vi "Find ROI Max Location v2.vi"(8 "error in (no error)":errorcluster, 9 "Source Image ROI Mask":T1, 10 "Source Image":T1, 11 "ROI Descriptor in":T2 {"Contours"."Type" items=["No Selection", "Point", "Line", "Rectangle", "Oval", "Polygon", "Freehand Region", "Annulus", "Unused2", "Unused3", "Broken Line", "Freehand Line", "Rotated Rectangle"]}) -> (0 "error out":errorcluster, 1 "Height":i32, 2 "Width":i32, 3 "ROI Mean Max Location":cluster{"X":i32, "Y":i32})   [LabVIEW 2021, in "Image.lvlib"]
uses:
  Image.lvlib
  <vilib>/vision/Image Controls.llb/IMAQ Image.ctl
  <vilib>/vision/EDVR.llb/IMAQ ImageToEDVR 2D U8.vi
  <vilib>/vision/EDVR.llb/IMAQ ImageToEDVR 2D I16.vi
  <vilib>/vision/EDVR.llb/IMAQ ImageToEDVR 2D SGL.vi
  <vilib>/vision/EDVR.llb/IMAQ ImageToEDVR 2D U16.vi
  <vilib>/vision/NI_Vision_Development_Module.lvlib
  Error/Error.lvlib
  Arrays/Arrays.lvlib
  Time/Time.lvlib
panel:
  out "elapsed (relative) seconds":dbl
  out "Waveform Chart":dbl[][](graph)
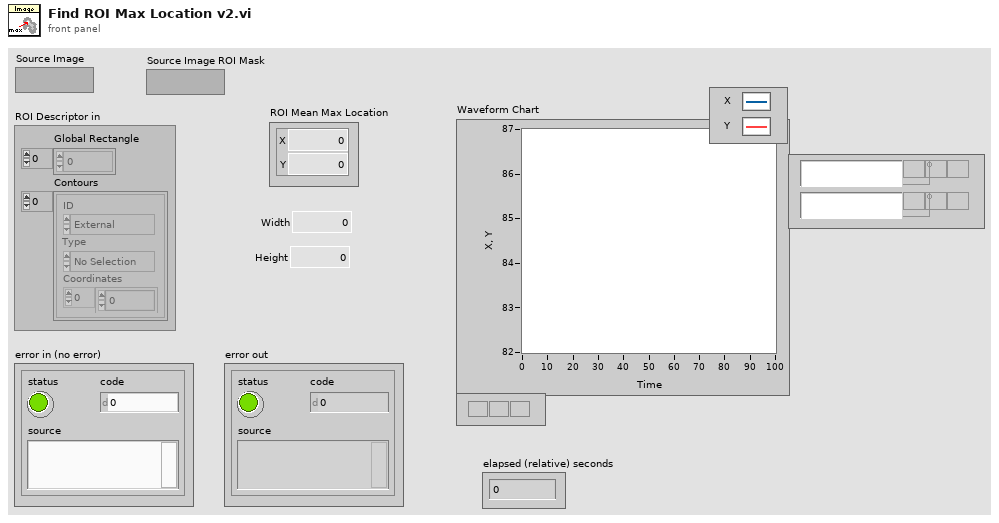
[diagram p1: front panel]
types:
  T1 = typedef "IMAQ Image.ctl" = refnum<image>
  T2 = typedef "ROI Descriptor" = cluster{"Global Rectangle":i32[], "Contours":cluster{"ID":enum32{"External", "Internal"}, "Type":u32, "Coordinates":i32[]}[]}
  T3 = typedef "Image Type" = u32
  T4 = cluster{"Numeric Control":i32, "Numeric Control":i32}[]
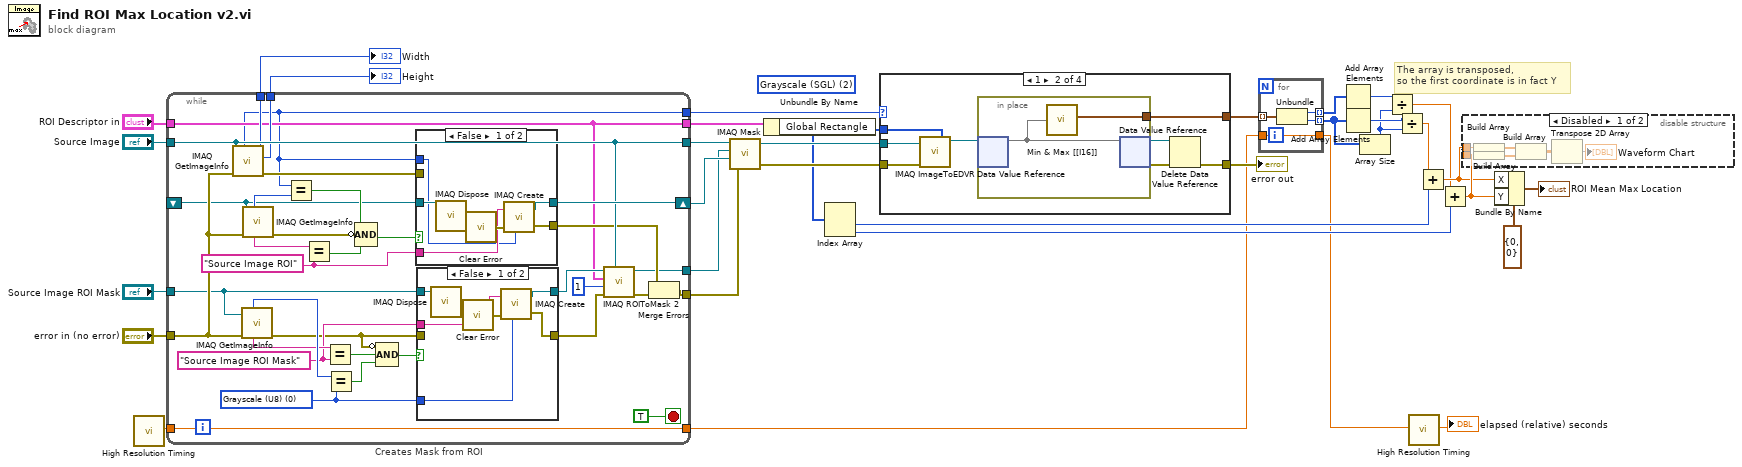
[diagram p0: block diagram]
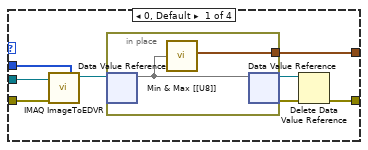
[diagram p3: hidden frame]
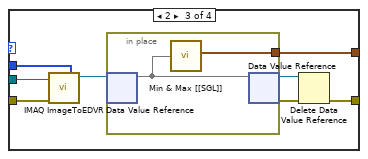
[diagram p4: hidden frame]
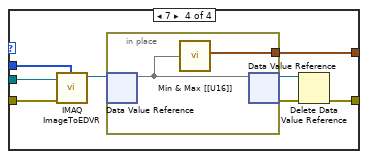
[diagram p5: hidden frame]
diagram:
  (unwired) T3 2 items=["Grayscale (U8)", "Grayscale (I16)", "Grayscale (SGL)", "Complex (CSG)", "RGB (U32)", "HSL (U32)", "RGB (U64)", "Grayscale (U16)"] ("Image Type")
  # "The array is transposed,\nso the first coordinate is in fact Y"
  n1 = call "High Resolution Timing.vi"() -> ("elapsed (relative) seconds"=w6:dbl)  [unwired: 17 in, 2 out]
  n2 = while "Creates Mask from ROI" {
    tunnel: "ROI Descriptor in" -> [w40]
    tunnel: "Source Image" -> [w47]
    tunnel: "error in (no error)" -> [w55]
    shift-right: [w49] -> w30
    shift-left: _ -> [w48]
    tunnel: [w47] -> w31
    tunnel: [w45] -> w29
    tunnel: [w42] -> w28
    tunnel: [w41] -> w27
    tunnel: [w40] -> w24
    tunnel: [w39] -> w23
    tunnel: w6 -> [w38]
    tunnel: [w38] -> w5
    tunnel: "Source Image ROI Mask" -> [w36]
    tunnel: [w35] -> w1
    stop <- TRUE stop-if-true
    w37 = "Source Image ROI" ("Image Name")
    w61 = "Source Image ROI Mask" ("Image Name")
    w60 = T3 0 items=["Grayscale (U8)", "Grayscale (I16)", "Grayscale (SGL)", "Complex (CSG)", "RGB (U32)", "HSL (U32)", "RGB (U64)", "Grayscale (U16)"] ("Image Type")
    n3 = call "IMAQ GetImageInfo"("error in (no error)"=w55, "Image"=w47) -> ("error out"=w43:errorcluster, "Y Resolution"=w41:i32, "X Resolution"=w42:i32, "Image Type"=w39:T3)  [unwired: 2 in, 4 out]
    n4 = call "IMAQ GetImageInfo"("error in (no error)"=w55, "Image"=w36) -> ("error out"=w58:errorcluster, "Image Name"=w66:string, "Image Type"=w67:T3)  [unwired: 2 in, 5 out]
    n5 = call "IMAQ GetImageInfo"("error in (no error)"=w55, "Image"=w48) -> ("error out"=w52:errorcluster, "Image Name"=w56:string, "Image Type"=w54:T3)  [unwired: 2 in, 5 out]
    n6 = Equal?(x=w39, y=w54) -> (x = y?=w51:bool)
    n7 = Equal?(x=w56, y=w37) -> (x = y?=w53:bool)
    n8 = Equal?(x=w66, y=w61) -> (x = y?=w64:bool)
    n9 = Equal?(x=w67, y=w60) -> (x = y?=w65:bool)
    n10 = Compound Arithmetic op=AND(w51, invert w52, w53) -> (w50:bool)
    n11 = Compound Arithmetic op=AND(invert w58, w64, w65) -> (w63:bool)
    n12 = case shown="False" w50 {
      tunnel: w48 -> [w75 w77]
      tunnel: w37 -> [w72 _]
      tunnel: w39 -> [w71 _]
      tunnel: [w70 w77] -> w49
      tunnel: [w69 w76] -> w44
      tunnel: w43 -> [_ w76]
      frame False {
        n13 = call "IMAQ Dispose"("Image"=w75) -> ("error out"=w74:errorcluster)  [unwired: 5 in]
        n14 = call "Clear Error.vi"("Error In"=w74) -> ("no Error Out"=w73:errorcluster)  [unwired: 8 in]
        n15 = call "IMAQ Create"("Image Name"=w72, "Image Type"=w71, "error in (no error)"=w73) -> ("New Image"=w70:T1, "error out"=w69:errorcluster)  [unwired: 2 in]
      }
      frame True {
      }
    }
    n16 = case shown="False" w63 {
      tunnel: w36 -> [w84 w86]
      tunnel: [w79 w86] -> w62
      tunnel: w61 -> [w81 _]
      tunnel: w60 -> [w80 _]
      tunnel: [w78 w85] -> w59
      tunnel: w58 -> [_ w85]
      frame False {
        n17 = call "IMAQ Dispose"("Image"=w84) -> ("error out"=w83:errorcluster)  [unwired: 5 in]
        n18 = call "Clear Error.vi"("Error In"=w83) -> ("no Error Out"=w82:errorcluster)  [unwired: 8 in]
        n19 = call "IMAQ Create"("Image Name"=w81, "Image Type"=w80, "error in (no error)"=w82) -> ("New Image"=w79:T1, "error out"=w78:errorcluster)  [unwired: 2 in]
      }
      frame True {
      }
    }
    n20 = call "IMAQ ROIToMask 2"("Image Model"=w47, "error in (no error)"=w59, "Filling Value (255)"=1, "ROI Descriptor"=w40, "Image"=w62) -> ("error out"=w46:errorcluster, "Image Out"=w35:T1)  [unwired: 4 in, 1 out]
    n21 = Merge Errors(w44, w46) -> (w45:errorcluster)
  }
  "Width" <- w28
  "Height" <- w27
  n22 = call "IMAQ Mask"("error in (no error)"=w29, "Image Dst"=w30, "Image Mask"=w1, "Image Src"=w31) -> ("error out"=w25:errorcluster, "Image Dst Out"=w26:T1)  [unwired: 1 in]
  n23 = Unbundle By Name(w24) -> ("Global Rectangle"=w22:i32[])
  n24 = Index Array(array=w22) -> (element #1=w21:i32, element #2=w20:i32)  [unwired: 2 in]
  n25 = case shown="1" w23 {
    tunnel: w26 -> [w94 w104 w114 w124]
    tunnel: w25 -> [w93 w103 w113 w123]
    tunnel: w22 -> [w92 w102 w112 w122]
    tunnel: [w90 w100 w110 w120] -> w15
    tunnel: [w87 w97 w107 w117] -> w7
    frame 0, Default {
      n26 = call-poly <vilib>:"IMAQ ImageToEDVR.vi"("Optional Rectangle"=w92, "error in (no error)"=w93, "Image"=w94) -> ("EDVR 2D U8"=w91:refnum<data-value>)  [unwired: 6 in, 2 out]
      n27 = in-place {
        in-place-border: [w96] -> w90
        n28 = in-place-dvr #1(w91) -> (w95:u8[][])  [unwired: 1 out]
        n29 = call "Min & Max [[U8]].vi"("Array"=w95) -> ("Array of Max Indices"=w96:T4)  [unwired: 4 in, 5 out]
        n30 = in-place-dvr #1(w95) -> (w89:refnum<data-value>, w88:errorcluster)
      }
      n31 = Delete Data Value Reference(data value reference=w89, error in=w88) -> (error out=w87:errorcluster)  [unwired: 1 out]
    }
    frame 1 {
      n32 = call-poly <vilib>:"IMAQ ImageToEDVR.vi"("Optional Rectangle"=w102, "error in (no error)"=w103, "Image"=w104) -> ("EDVR 2D I16"=w101:refnum<data-value>)  [unwired: 6 in, 2 out]
      n33 = in-place {
        in-place-border: [w106] -> w100
        n34 = in-place-dvr #2(w101) -> (w105:i16[][])  [unwired: 1 out]
        n35 = call "Min & Max [[I16]].vi"("Array"=w105) -> ("Array of Max Indices"=w106:T4)  [unwired: 4 in, 5 out]
        n36 = in-place-dvr #2(w105) -> (w99:refnum<data-value>, w98:errorcluster)
      }
      n37 = Delete Data Value Reference(data value reference=w99, error in=w98) -> (error out=w97:errorcluster)  [unwired: 1 out]
    }
    frame 2 {
      n38 = call-poly <vilib>:"IMAQ ImageToEDVR.vi"("Optional Rectangle"=w112, "error in (no error)"=w113, "Image"=w114) -> ("EDVR 2D SGL"=w111:refnum<data-value>)  [unwired: 6 in, 2 out]
      n39 = in-place {
        in-place-border: [w116] -> w110
        n40 = in-place-dvr #3(w111) -> (w115:sgl[][])  [unwired: 1 out]
        n41 = call "Min & Max [[SGL]].vi"("Array"=w115) -> ("Array of Max Indices"=w116:T4)  [unwired: 4 in, 5 out]
        n42 = in-place-dvr #3(w115) -> (w109:refnum<data-value>, w108:errorcluster)
      }
      n43 = Delete Data Value Reference(data value reference=w109, error in=w108) -> (error out=w107:errorcluster)  [unwired: 1 out]
    }
    frame 7 {
      n44 = call-poly <vilib>:"IMAQ ImageToEDVR.vi"("Optional Rectangle"=w122, "error out"=w123, "Image"=w124) -> ("EDVR 2D U16"=w121:refnum<data-value>)  [unwired: 6 in, 2 out]
      n45 = in-place {
        in-place-border: [w126] -> w120
        n46 = in-place-dvr #4(w121) -> (w125:u16[][])  [unwired: 1 out]
        n47 = call "Min & Max [[U16]].vi"("Array"=w125) -> ("Array of Max Indices"=w126:T4)  [unwired: 4 in, 5 out]
        n48 = in-place-dvr #4(w125) -> (w119:refnum<data-value>, w118:errorcluster)
      }
      n49 = Delete Data Value Reference(data value reference=w119, error in=w118) -> (error out=w117:errorcluster)  [unwired: 1 out]
    }
  }
  "error out" <- w7
  n50 = for {
    tunnel: w15 -> [w130] mode=indexing
    tunnel: [w129] -> w14 mode=indexing
    tunnel: [w128] -> w13 mode=indexing
    tunnel: [w127] -> w4
    tunnel: w5 -> [w127]
    n51 = Unbundle(w130) -> ("Numeric Control"=w129:i32, "Numeric Control"=w128:i32)
  }
  n52 = Add Array Elements(numeric array=w14) -> (sum=w12:i32)
  n53 = Add Array Elements(numeric array=w13) -> (sum=w11:i32)
  n54 = Array Size(array=w13) -> (size(s)=w10:i32)
  n55 = Divide(x=w12, y=w10) -> (x/y=w9:dbl)
  n56 = Divide(x=w11, y=w10) -> (x/y=w8:dbl)
  n57 = call "High Resolution Timing.vi"("relative seconds (NaN)"=w4) -> ("elapsed (relative) seconds"=→"elapsed (relative) seconds":dbl)  [unwired: 16 in, 2 out]
  n58 = Add(x=w8, y=w21) -> (x+y=w16:dbl)
  n59 = Add(x=w9, y=w20) -> (x+y=w17:dbl)
  n60 = disable-structure shown="Disabled" {
    disable-tunnel: w17 -> [w132 _]
    disable-tunnel: w16 -> [w131 _]
    frame Disabled {
      n61 = Build Array(w131) -> (w136:dbl[])
      n62 = Build Array(w132) -> (w135:dbl[])
      n63 = Build Array(w136, w135) -> (w134:dbl[][])
      n64 = Transpose 2D Array(2D array=w134) -> (transposed array=→"Waveform Chart":dbl[][])
    }
    frame Enabled {
    }
  }
  n65 = Bundle By Name(cluster=cluster{"X":i32, "Y":i32} {"X"=0, "Y"=0} ("ROI Center"), "X"=w16, "Y"=w17) -> (→"ROI Mean Max Location":cluster{"X":i32, "Y":i32})
